vi "Get VI Refnum.vi"(8 "error in (no error)":errorcluster, 11 "Coca Actors in":refnum<class "Coca Actors.lvclass">) -> (0 "error out":errorcluster, 2 "VI Refnum":refnum<vi>, 3 "Coca Actors out":refnum<class "Coca Actors.lvclass">)   [LabVIEW 2020, in "Coca Actors.lvlib" / "Coca Actors.lvclass"]
uses:
  Coca Actors.lvclass
  Coca Actors.lvclass/Coca Actors.ctl
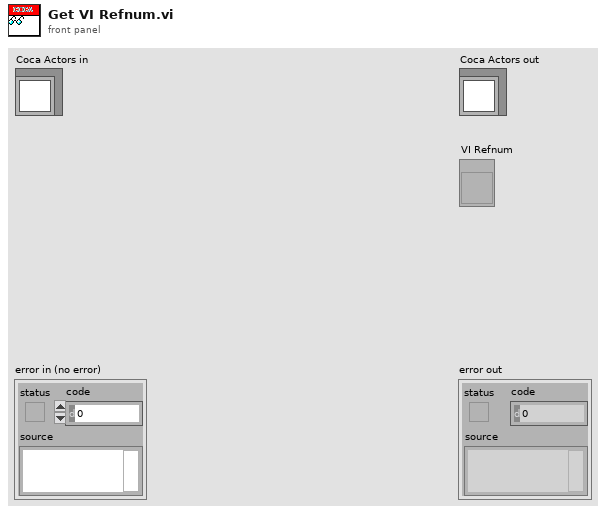
[diagram p1: front panel]
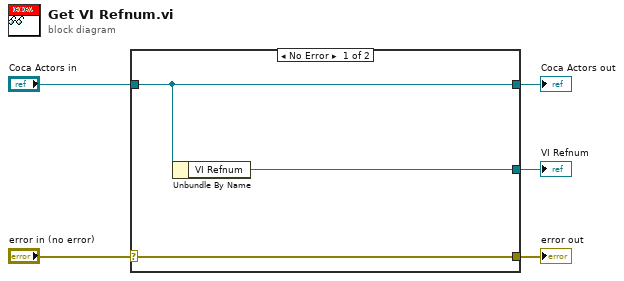
[diagram p0: block diagram]
diagram:
  n1 = case shown="No Error" "error in (no error)" {
    selector: "error in (no error)" -> [w8 w9]
    tunnel: [w8 w9] -> w4
    tunnel: [w7 w10] -> w2
    tunnel: "Coca Actors in" -> [w7 w10]
    tunnel: [w6 _] -> w1
    frame No Error {
      n2 = Unbundle By Name(w7) -> ("VI Refnum"=w6:refnum<vi>)
    }
    frame Error {
    }
  }
  "error out" <- w4
  "Coca Actors out" <- w2
  "VI Refnum" <- w1
